vi "Find Value.vi"(8 "error in":errorcluster, 9 "Path Style":enum16{"JSONPath", "XPath"}(ring), 10 "Attribute":string, 11 "DOM":refnum<k20>) -> (0 "error out":errorcluster, 3 "Value":string)   [LabVIEW 2019, in "Configuration.lvlib" / "Config from XML.lvclass"]
uses:
  Config from XML.lvclass
  Config from XML.lvclass/Config from XML.ctl
  <vilib>/xml/NI_XML.lvlib
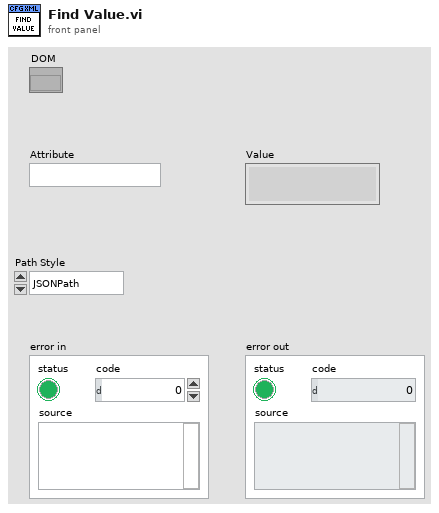
[diagram p1: front panel]
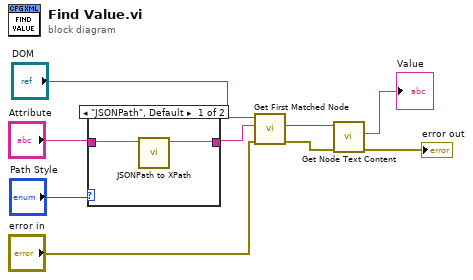
[diagram p0: block diagram]
diagram:
  n1 = case shown="\"JSONPath\", Default" "Path Style" {
    tunnel: "Attribute" -> [w11 w12]
    tunnel: [w10 w12] -> w7
    frame "JSONPath", Default {
      n2 = call "JSONPath to XPath.vi"("JSONPath"=w11) -> ("XPath"=w10:string)  [unwired: 10 in]
    }
    frame "XPath" {
    }
  }
  n3 = call <vilib>:"Get First Matched Node.vi"("error in (no error)"="error in", "XPath expression"=w7, "node in"="DOM") -> ("error out"=w3:errorcluster, "node result"=w4:refnum<k20>)  [unwired: 6 in, 1 out]
  n4 = call <vilib>:"Get Node Text Content.vi"("error in (no error)"=w3, "node in"=w4) -> ("error out"=→"error out":errorcluster, "node text"=→"Value":string)  [unwired: 7 in, 1 out]
